vi "Bar chart.vi"() -> ()   [LabVIEW 2019]
uses:
  <vilib>/Utility/miscctls.llb/LVAnnotationListTypeDef.ctl
panel:
  out "Array":i32[](array[numeric])
  out "XY Graph":cluster{i32[], i32[]}(graph)
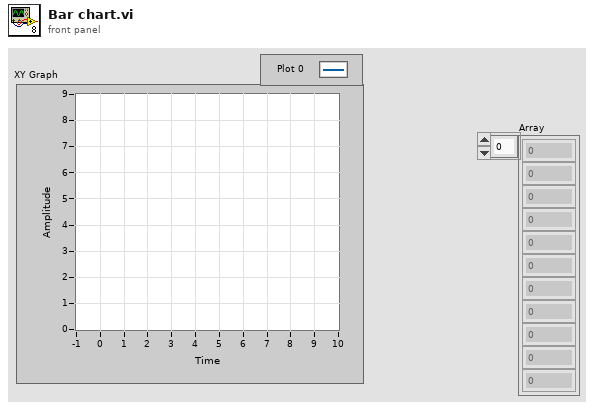
[diagram p1: front panel]
types:
  T1 = typedef "LVAnnotationListTypeDef.ctl" = cluster{"Name":string, "Color":u32, "Style":u8, "Point Style":u8, "Name Visible":bool, "Allow Drag":bool, "Annotation Mode":u32, "Plot":i32, "Index":i32, "Position":cluster{"X":dbl, "Y":dbl}, "X Scale":u32, "Y Scale":u32, "Show Arrow":bool, "Lock Name":bool, "Plot Area":i32, "Label Offset":cluster{"X":dbl, "Y":dbl}}[]
  T2 = cluster{"Name":string, "Color":u32, "Style":u8, "Point Style":u8, "Name Visible":bool, "Allow Drag":bool, "Annotation Mode":u32, "Plot":i32, "Index":i32, "Position":cluster{"X":dbl, "Y":dbl}, "X Scale":u32, "Y Scale":u32, "Show Arrow":bool, "Lock Name":bool, "Plot Area":i32, "Label Offset":cluster{"X":dbl, "Y":dbl}}
  T3 = cluster{"Name":string, "Color":u32, "Style":u8, "Point Style":u8, "Name Visible":bool, "Allow Drag":bool, "Annotation Mode":u32, "Plot":i32, "Index":i32, "Position":cluster{"X":dbl, "Y":dbl}, "X Scale":u32, "Y Scale":u32, "Show Arrow":bool, "Lock Name":bool, "Plot Area":i32, "Label Offset":cluster{"X":dbl, "Y":dbl}}[]
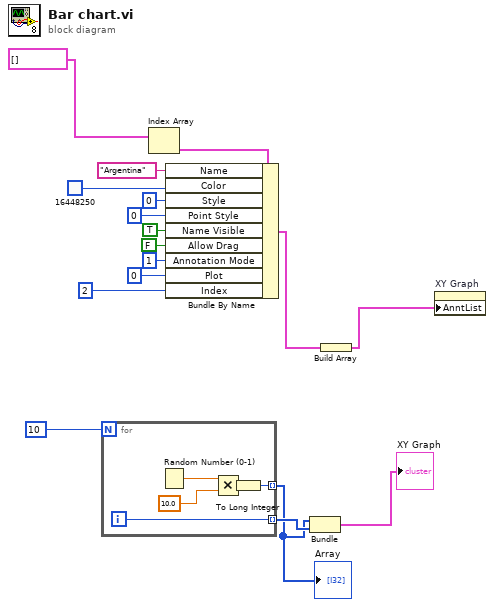
[diagram p0: block diagram]
diagram:
  n1 = for {
    N: 10 -> [_]
    tunnel: [w18] -> w14 mode=indexing
    tunnel: [w19] -> w15 mode=indexing
    i -> [w19]
    n2 = Random Number (0-1)() -> (number: 0 to 1=w22:dbl)
    n3 = Multiply(x=w22, y=10.0) -> (x*y=w20:dbl)
    n4 = To Long Integer(number=w20) -> (32bit integer=w18:i32)
  }
  "Array" <- w14
  n5 = Index Array(array=T1 [] ("Annotation List")) -> (element=w12:T2)  [unwired: 1 in]
  n6 = Bundle By Name(cluster=w12, "Name"="Argentina", "Color"=u32 16448250, "Style"=u8 0, "Point Style"=u8 0, "Name Visible"=TRUE, "Allow Drag"=FALSE, "Annotation Mode"=u32 1, "Plot"=0, "Index"=2) -> (w11:T2)
  n7 = Bundle(w14, w15) -> (→"XY Graph":cluster{i32[], i32[]})  [unwired: 1 in]
  n8 = Build Array(w11) -> (w10:T3)
  n9 = property on="XY Graph" class="XYGraph (strict)"("AnntList"=w10) -> ()  [unwired: 2 in, 2 out]
